vi "vector_to_pose.vi"(4 "Angle unit":enum16{"Radians", "Degrees"}(ring)=enum."Degrees", 6 "Translation scale":dbl=1000.0 format="%#_6p", 11 "Pose vector":dbl[](array[numeric])) -> (3 "Pose":T1)   [LabVIEW 2013]
uses:
  <vilib>/Analysis/Matrix/Datatypes/RealMatrix.ctl
  <vilib>/Analysis/coordinate.llb/Euler Rotation Order.ctl
  <vilib>/Analysis/Matrix/Numeric/Conversions/Array To Matrix - RA.vi
  <vilib>/Analysis/Matrix/NI_Matrix.lvlib
  <vilib>/Analysis/NI_AALPro.lvlib
panel:
  # "Multiply XYZ by this."
  # "Rotations in degrees or radians?"
  # "Convert pose represented as X Y Z Rx Ry Rz into transform matrix."
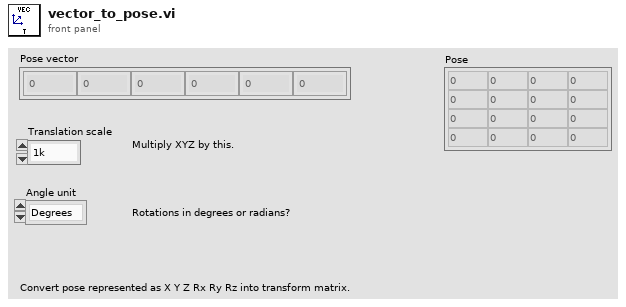
[diagram p1: front panel]
types:
  T1 = typedef "NI_Matrix.lvlib/RealMatrix.ctl" = dbl[][]
  T2 = typedef "NI_AALPro.lvlib/Euler Rotation Order.ctl" = u16
  T3 = cluster{"Pose vector[0]":dbl, "Pose vector[1]":dbl, "Pose vector[2]":dbl}
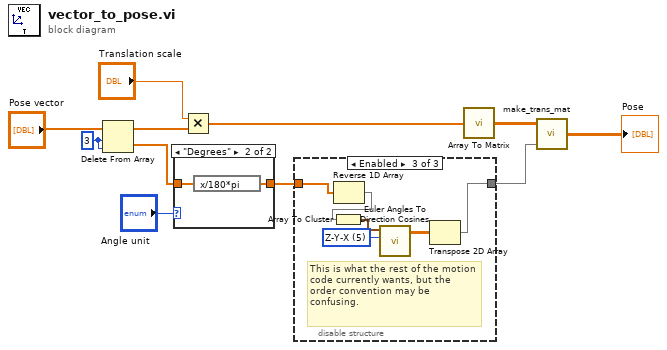
[diagram p0: block diagram]
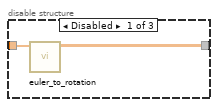
[diagram p2: hidden frame]
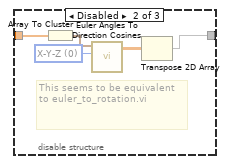
[diagram p3: hidden frame]
diagram:
  w8 = 3 ("length")
  n1 = Delete From Array(array="Pose vector", length=w8, index=w8) -> (deleted portion=w2:dbl[], array with subset deleted=w6:dbl[])
  n2 = case shown="\"Degrees\"" "Angle unit" {
    tunnel: w2 -> [w12 w14]
    tunnel: [w12 w13] -> w1
    frame "Radians", Default {
    }
    frame "Degrees" {
      n3 = expression code="x/180*pi"(w14) -> (w13:dbl[])
    }
  }
  n4 = Multiply(x="Translation scale", y=w6) -> (x*y=w5:dbl[])
  n5 = disable-structure shown="Enabled" {
    disable-tunnel: [w16 w17 w24] -> w10
    disable-tunnel: w1 -> [w15 w19 w23]
    frame Disabled {
      n6 = call "euler_to_rotation.vi"("Theta XYZ"=w15) -> ("Rotation"=w16:T1)  [unwired: 10 in]
    }
    frame Disabled {
      w20 = T2 0 items=["X-Y-Z", "X-Z-Y", "Y-X-Z", "Y-Z-X", "Z-X-Y", "Z-Y-X", "X-Y-X", "X-Z-X", "Y-X-Y", "Y-Z-Y", "Z-X-Z", "Z-Y-Z"] ("rotation order")
      # "This seems to be equivalent to euler_to_rotation.vi"
      n7 = Array To Cluster(array=w19) -> (cluster=w21:T3)
      n8 = call <vilib>:"Euler Angles To Direction Cosines.vi"("rotation order"=w20, "Euler Angles"=w21) -> ("Direction Cosines"=w18:dbl[][])  [unwired: 8 in, 1 out]
      n9 = Transpose 2D Array(2D array=w18) -> (transposed array=w17:dbl[][])
    }
    frame Enabled {
      w26 = T2 5 items=["X-Y-Z", "X-Z-Y", "Y-X-Z", "Y-Z-X", "Z-X-Y", "Z-Y-X", "X-Y-X", "X-Z-X", "Y-X-Y", "Y-Z-Y", "Z-X-Z", "Z-Y-Z"] ("rotation order")
      # "This is what the rest of the motion code currently wants, but the order convention may be confusing."
      n10 = Reverse 1D Array(array=w23) -> (reversed array=w22:dbl[])
      n11 = Array To Cluster(array=w22) -> (cluster=w27:cluster{"[0]":dbl, "[1]":dbl, "[2]":dbl})
      n12 = call <vilib>:"Euler Angles To Direction Cosines.vi"("rotation order"=w26, "Euler Angles"=w27) -> ("Direction Cosines"=w25:dbl[][])  [unwired: 8 in, 1 out]
      n13 = Transpose 2D Array(2D array=w25) -> (transposed array=w24:dbl[][])
    }
  }
  n14 = call-poly <vilib>:"Array To Matrix.vi"("Real 1D Array"=w5) -> ("Real Matrix (Column Vector)"=w9:T1)
  n15 = call "make_trans_mat.vi"("Rotation"=w10, "Translation"=w9) -> ("Transform"=→"Pose":T1)  [unwired: 3 in]
